vi "DriveStraight.vi"(11 "Angle":dbl) -> (3 "Turn":dbl)   [LabVIEW 2016]
uses:
  Robot Global Data.vi
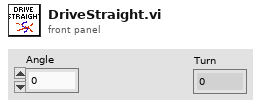
[diagram p1: front panel]
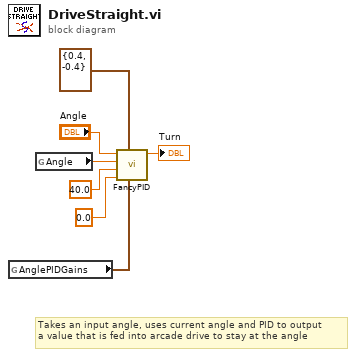
[diagram p0: block diagram]
diagram:
  # "Takes an input angle, uses current angle and PID to output\na value that is fed into arcade drive to stay at the angle"
  n1 = global read "Robot Global Data.vi" "AnglePIDGains"() -> (w1:cluster{" P":dbl, "I":dbl, "D":dbl})
  n2 = global read "Robot Global Data.vi" "Angle"() -> (w6:dbl)
  n3 = call "FancyPID.vi"("Gains"=w1, "Range"=cluster{"output high":dbl, "output low":dbl} {"output high"=0.4, "output low"=-0.4}, "Disable Range"=0.0, "Integral Range"=40.0, "Process variable"=w6, "Setpoint"="Angle") -> ("output"=→"Turn":dbl)  [unwired: 5 in]
